vi "Channel_ToXML.vi"(8 "error in (no error)":errorcluster, 11 "Channel in":refnum<class "Channel.lvclass">) -> (0 "error out":errorcluster, 2 "XML String":string, 3 "Channel out":refnum<class "Channel.lvclass">)   [LabVIEW 2023, in "Channel.lvclass"]
doc: "Export the current channel definition to XML."
uses:
  Channel.lvclass
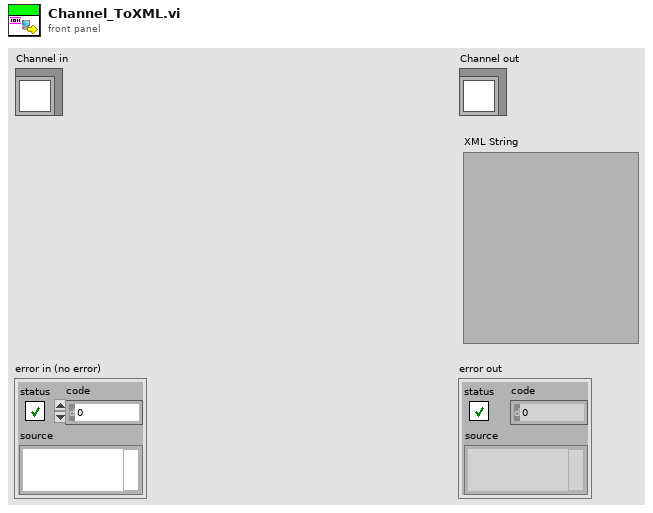
[diagram p1: front panel]
types:
  T1 = typedef "ChannelAsCluster.ctl" = cluster{"Name":string, "Data Reference":T2, "Wfm?":bool, "Decimation":i32, "Current Value":dbl, "Meta Data":T3[], "WfmPath":string}
  T2 = typedef "Custom Device API.lvlib/Data Reference.ctl" = i32
  T3 = typedef "Meta Data.ctl" = cluster{"Key":string, "Value":string}
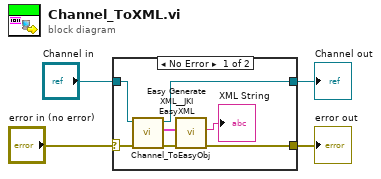
[diagram p0: block diagram]
diagram:
  n1 = case shown="No Error" "error in (no error)" {
    selector: "error in (no error)" -> [w8 w13]
    tunnel: [w10 w13] -> w3
    tunnel: [w6 w12] -> w1
    tunnel: "Channel in" -> [w9 w12]
    frame No Error {
      n2 = call-dynamic "Channel_ToEasyObj.vi"("error in (no error)"=w8, "Channel in"=w9) -> ("error out"=w5:errorcluster, "output cluster"=w7:T1, "Channel out"=w6:refnum<class "Channel.lvclass">)  [unwired: 7 in]
      n3 = call <vilib>:"Easy Generate XML__JKI EasyXML.vi"("error in (no error)"=w5, "LabVIEW Data"=w7) -> ("error out"=w10:errorcluster, "XML String"=→"XML String":string)  [unwired: 8 in]
    }
    frame Error {
    }
  }
  "error out" <- w3
  "Channel out" <- w1
